vi "Load Expense Summaries.vi"(8 "error in (no error)":errorcluster, 10 "SQL Date":string, 11 "Database in":refnum<class "Database.lvclass">) -> (0 "error out":errorcluster, 2 "Bdgt Values":string[][](array[string]), 3 "Database out":refnum<class "Database.lvclass">)   [LabVIEW 2018, in "Database.lvclass"]
uses:
  Database.lvclass
  Expense Summary/Expense Summary.lvclass
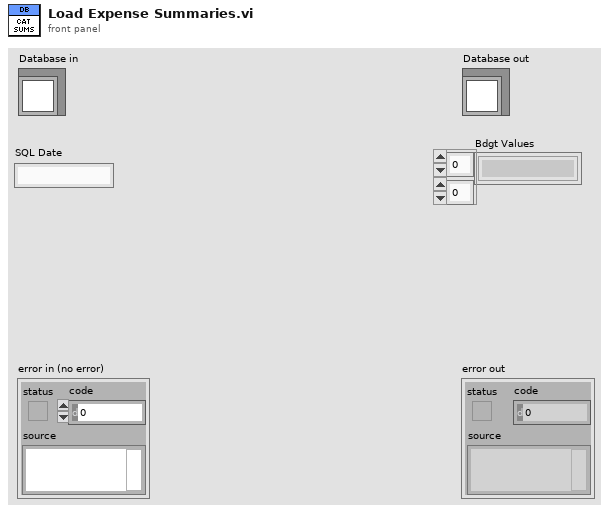
[diagram p1: front panel]
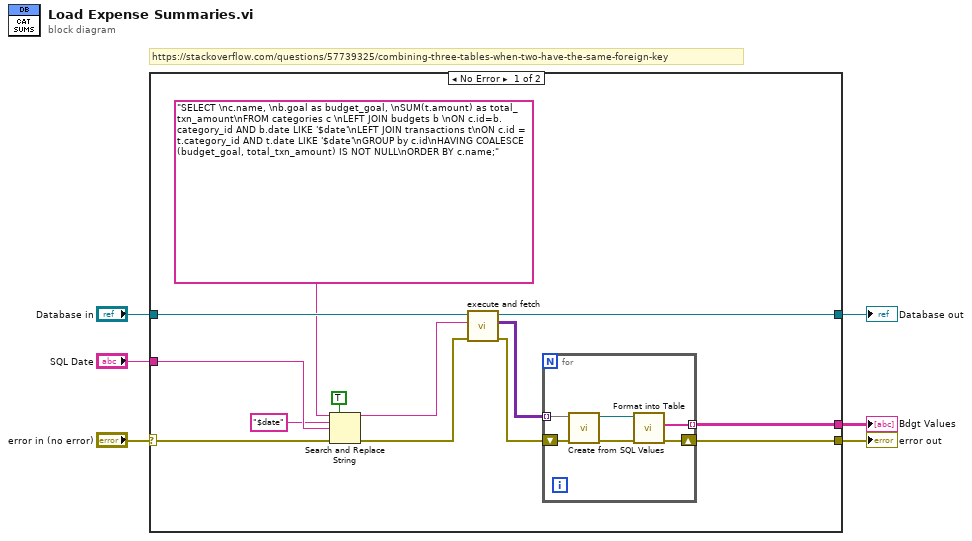
[diagram p0: block diagram]
diagram:
  # "https://stackoverflow.com/questions/57739325/combining-three-tables-when-two-have-the-same-foreign-key"
  n1 = case shown="No Error" "error in (no error)" {
    selector: "error in (no error)" -> [w14 w26]
    tunnel: [w17 w27] -> w6
    tunnel: "Database in" -> [w16 w27]
    tunnel: [w15 w26] -> w4
    tunnel: "SQL Date" -> [w12 _]
    tunnel: [w7 _] -> w2
    frame No Error {
      n2 = Search and Replace String(replace all?=TRUE ("replace all? (F)"), input string="SELECT \nc.name, \nb.goal as budget_goal, \nSUM(t.amount) as total_txn_amount\nFROM categories c \nLEFT JOIN budgets b \nON c.id=b.category_id AND b.date LIKE '$date'\nLEFT JOIN transactions t\nON c.id = t.category_id AND t.date LIKE '$date'\nGROUP by c.id\nHAVING COALESCE (budget_goal, total_txn_amount) IS NOT NULL\nORDER BY c.name;", search string="$date", replace string=w12, error in=w14) -> (result string=w9:string, error out=w13:errorcluster)  [unwired: 3 in, 2 out]
      n3 = call "execute and fetch.vi"("error in (no error)"=w13, "SQL query"=w9, "Database in"=w16) -> ("error out"=w18:errorcluster, "recordset data"=w19:variant[][], "Database out"=w17:refnum<class "Database.lvclass">)  [unwired: 5 in, 1 out]
      n4 = for {
        tunnel: w19 -> [w24] mode=indexing
        shift-right: [w22] -> w15
        shift-left: w18 -> [w25]
        tunnel: [w20] -> w7 mode=indexing
        n5 = call "Create from SQL Values.vi"("error in (no error)"=w25, "recordset data"=w24) -> ("error out"=w23:errorcluster, "Expense Summary out"=w21:refnum<class "Expense Summary.lvclass">)  [unwired: 8 in]
        n6 = call "Format into Table.vi"("error in (no error)"=w23, "Expense Summary in"=w21) -> ("error out"=w22:errorcluster, "Summary Values"=w20:string[])  [unwired: 7 in, 1 out]
      }
    }
    frame Error {
    }
  }
  "error out" <- w4
  "Database out" <- w6
  "Bdgt Values" <- w2
